vi "Read Array.vi"(8 "error in (no error)":errorcluster, 11 "Controller Array in":refnum<class "Controller Array.lvclass">) -> (0 "error out":errorcluster, 2 "Array":refnum<class "Generic Plugin.lvclass">[](array[class]), 3 "Controller Array out":refnum<class "Controller Array.lvclass">)   [LabVIEW 2020, in "Controller Array.lvclass"]
uses:
  Controller Array.lvclass
  Controller/Generic Plugin.lvclass
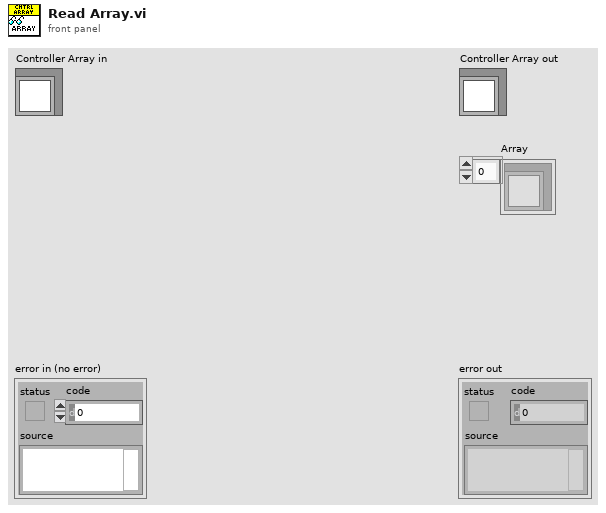
[diagram p1: front panel]
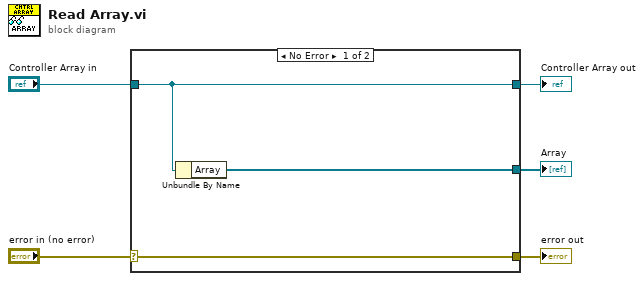
[diagram p0: block diagram]
diagram:
  n1 = case shown="No Error" "error in (no error)" {
    selector: "error in (no error)" -> [w8 w9]
    tunnel: [w8 w9] -> w4
    tunnel: [w7 w10] -> w2
    tunnel: "Controller Array in" -> [w7 w10]
    tunnel: [w6 _] -> w1
    frame No Error {
      n2 = Unbundle By Name(w7) -> ("Array"=w6:refnum<class "Generic Plugin.lvclass">[])
    }
    frame Error {
    }
  }
  "error out" <- w4
  "Controller Array out" <- w2
  "Array" <- w1
